vi "Set Row Tag.vi"(8 "error in":errorcluster, 9 "object":variant, 10 "Row Index":i32, 11 "SourceGrid in":refnum<class "SourceGrid.lvclass">) -> (0 "error out":errorcluster, 3 "SourceGrid out":refnum<class "SourceGrid.lvclass">)   [LabVIEW 2024, in "SourceGrid.lvlib" / "SourceGrid.lvclass"]
uses:
  SourceGrid.lvclass
  SourceGrid.lvclass/SourceGrid.ctl
  D:/git/Sourcegrid-LabVIEW/dll/SourceGrid.dll
  dll/SourceGrid.dll
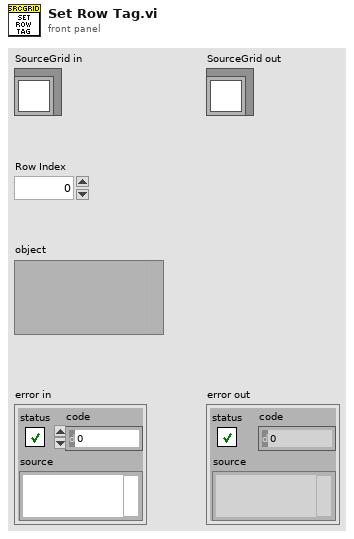
[diagram p1: front panel]
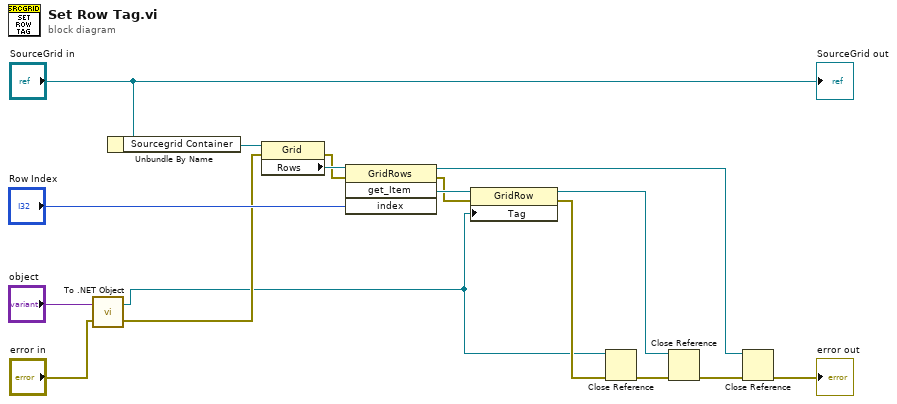
[diagram p0: block diagram]
diagram:
  n1 = call <vilib>:"To .NET Object.vi"("error in (no error)"="error in", "anything"="object") -> ("error out"=w5:errorcluster, ".NET object"=w1:refnum<k24>)
  n2 = Unbundle By Name("SourceGrid in") -> ("Sourcegrid Container"=w16:refnum<k24>)
  n3 = property class="Grid"(reference=w16, error in=w5) -> (error out=w4:errorcluster, "Rows"=w13:refnum<k24>)  [unwired: 1 out]
  n4 = invoke class="GridRows" method="get_Item"(reference=w13, error in=w4, "index"="Row Index") -> (reference out=w6:refnum<k24>, error out=w3:errorcluster, "get_Item"=w11:refnum<k24>)  [unwired: 1 in, 1 out]
  n5 = property class="GridRow"(reference=w11, error in=w3, "Tag"=w1) -> (reference out=w8:refnum<k24>, error out=w9:errorcluster)
  n6 = Close Reference(reference=w1, error in (no error)=w9) -> (error out=w2:errorcluster)
  n7 = Close Reference(reference=w8, error in (no error)=w2) -> (error out=w10:errorcluster)
  n8 = Close Reference(reference=w6, error in (no error)=w10) -> (error out=→"error out":errorcluster)
  "SourceGrid out" <- "SourceGrid in"
